vi "CThread Wait For Initialization.vi"(4 "Timeout (300 ms)":u32=300) -> (1 "Active?":bool)   [LabVIEW 2012, in "CThread.lvlib"]
uses:
  CThread.lvlib
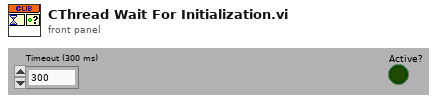
[diagram p1: front panel]
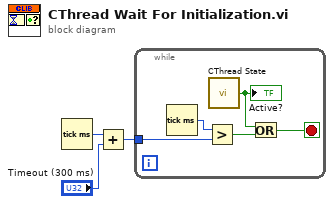
[diagram p0: block diagram]
diagram:
  n1 = Tick Count (ms)() -> (millisecond timer value=w3:u32)
  n2 = Add(x=w3, y="Timeout (300 ms)") -> (x+y=w1:u32)
  n3 = while {
    tunnel: w1 -> [w6]
    stop <- w8 stop-if-true
    n4 = Tick Count (ms)() -> (millisecond timer value=w5:u32)
    n5 = Greater?(x=w5, y=w6) -> (0:w4:bool)
    n6 = call "CThread State.vi"() -> ("Active?"=w7:bool)  [unwired: 4 in, 1 out]
    "Active?" <- w7
    n7 = Or(x=w7, y=w4) -> (x .or. y?=w8:bool)
  }
